vi "State Triggered Reason.vi"(9 "Source CSM":string, 11 "Additional Information":T1) -> (1 "Reason":T2, 2 "Source CSM (dup)":string, 3 "Additional Information (dup)":T1)   [LabVIEW 2017, in "Communicable State Machine.lvlib"]
uses:
  Communicable State Machine.lvlib
  _Support/Typedef/_CSM_Response Source Message.ctl
  _Support/Typedef/_CSM_STATE_CALL_REASON.ctl
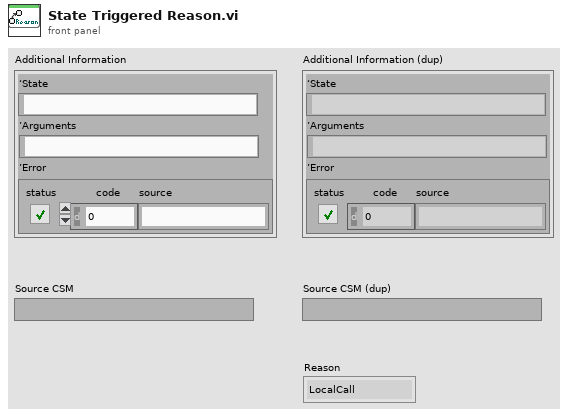
[diagram p1: front panel]
types:
  T1 = typedef "Communicable State Machine.lvlib/_CSM_Response Source Message.ctl" = cluster{"‘State":string, "’Arguments":string, "’Error":errorcluster}
  T2 = typedef "Communicable State Machine.lvlib/_CSM_STATE_CALL_REASON.ctl" = enum16{"LocalCall", "Message", "Broadcast"}
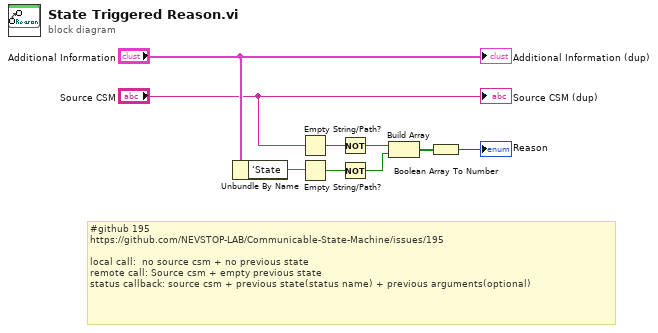
[diagram p0: block diagram]
diagram:
  # "#github 195\nhttps://github.com/NEVSTOP-LAB/Communicable-State-Machine/issues/195\n\nlocal call:  no source csm + no previous state\nremote call: Source csm + empty previous state\nstatus callback: source csm + previous state(status name) + previous arguments(optional)"
  n1 = Unbundle By Name("Additional Information") -> ("‘State"=w8:string)
  n2 = Empty String/Path?(string/path="Source CSM") -> (empty?=w5:bool)
  n3 = Empty String/Path?(string/path=w8) -> (empty?=w6:bool)
  n4 = Not(x=w5) -> (.not. x?=w2:bool)
  n5 = Not(x=w6) -> (.not. x?=w1:bool)
  n6 = Build Array(w2, w1) -> (w4:bool[])
  n7 = Boolean Array To Number(Boolean array=w4) -> (number=→"Reason":u32)
  "Source CSM (dup)" <- "Source CSM"
  "Additional Information (dup)" <- "Additional Information"
